vi "Stop_Main_FGV.vi"(7 "Command":enum16{"set", "get", "init"}(ring), 11 "Stop":bool) -> (3 "Stop out":bool)   [LabVIEW 2020]
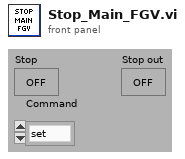
[diagram p1: front panel]
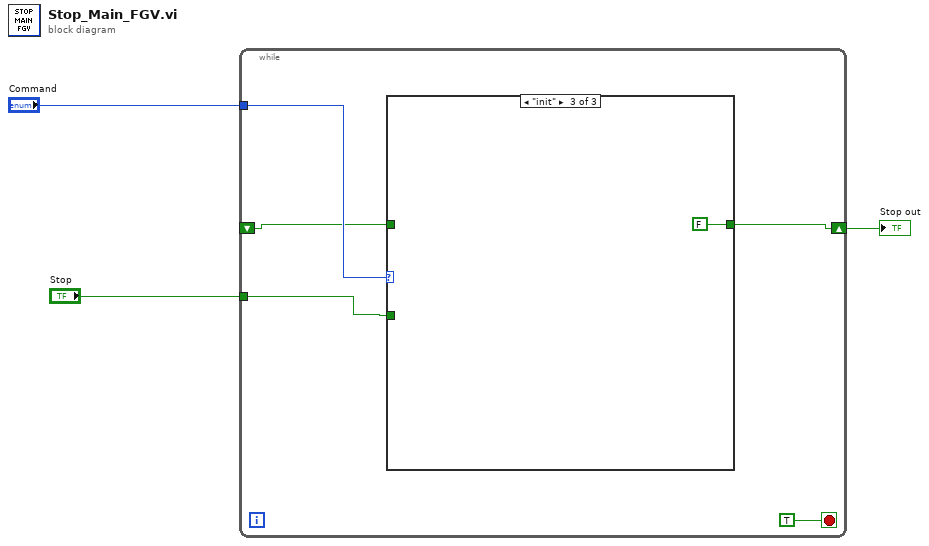
[diagram p0: block diagram]
diagram:
  n1 = while {
    tunnel: "Stop" -> [w7]
    shift-right: [w5] -> w3
    shift-left: _ -> [w4]
    tunnel: "Command" -> [w6]
    stop <- TRUE stop-if-true
    n2 = case shown="\"init\"" w6 {
      tunnel: w7 -> [w9 _ _]
      tunnel: [w9 w10 FALSE ("clear buffer")] -> w5
      tunnel: w4 -> [_ w10 _]
      frame "set", Default {
      }
      frame "get" {
      }
      frame "init" {
      }
    }
  }
  "Stop out" <- w3
